vi "PH_AxisGUI_BaseClass.PC Relative Move.vi"(0 "i ref in":refnum<vi>, 2 "Axis":i32=-1, 4 "direction":T1, 5 "error in":errorcluster) -> (14 "i ref out":refnum<vi>, 19 "error out":errorcluster)   [LabVIEW 2014, in "PH_AxisGUI_BaseClass.lvlib"]
doc: "This VI acts on an axis."
uses:
  PH_AxisGUI_BaseClass.lvlib
  PH_Stepmotor_BaseClass/PH_Stepmotor_BaseClass.Axis Direction.ctl
  PH_Stepmotor_BaseClass/PH_Stepmotor_BaseClass.lvlib
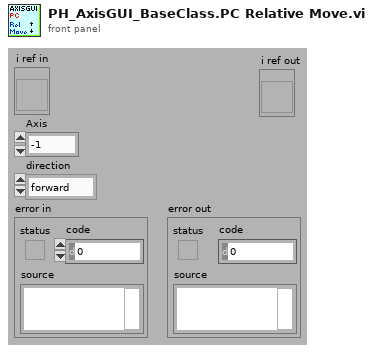
[diagram p1: front panel]
types:
  T1 = typedef "PH_Stepmotor_BaseClass.lvlib/PH_Stepmotor_BaseClass.Axis Direction.ctl" = enum16{"forward", "backward"}
  T2 = typedef "PH_Stepmotor_BaseClass.lvlib/PH_Stepmotor_BaseClass.Axis Address.ctl" = cluster{"Instance":string, "Motor Nr":i32}
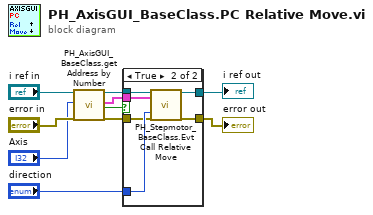
[diagram p0: block diagram]
diagram:
  n1 = call "PH_AxisGUI_BaseClass.get Address by Number.vi"("VI in"="i ref in", "Axis"="Axis", "error in (no error)"="error in") -> ("VI out"=w5:refnum<vi>, "Address"=w3:T2, "Axis exists and is not moving?"=w2:bool, "error out"=w4:errorcluster)  [unwired: 12 in, 1 out]
  n2 = case "Axis exists?" shown="True" w2 {
    tunnel: "direction" -> [_ w18]
    tunnel: [w12 w14] -> w7
    tunnel: [w11 w13] -> w6
    tunnel: w5 -> [w12 w17]
    tunnel: w4 -> [w11 w16]
    tunnel: w3 -> [_ w15]
    frame False {
    }
    frame True {
      n3 = call "PH_Stepmotor_BaseClass.Evt Call Relative Move.vi"("i ref in"=w17, "Address"=w15, "direction"=w18, "error in"=w16) -> ("i ref out"=w14:refnum<vi>, "error out"=w13:errorcluster)  [unwired: 14 in]
    }
  }
  "error out" <- w6
  "i ref out" <- w7
